vi "createColorProjections.vi"(4 "xyz order":bool, 6 "max values":T2={"xy max"={"r max"=-1.0, "g max"=-1.0, "b max"=-1.0}, "xz max"={"r max"=-1.0, "g max"=-1.0, "b max"=-1.0}, "zy max"={"r max"=-1.0, "g max"=-1.0, "b max"=-1.0}}, 7 "display channels":cluster{"CH0":bool, "CH1":bool}, 8 "error in (no error)":errorcluster, 9 "spilt ff/fb":bool, 10 "color ims":cluster{"xy im":T3, "xz im":T3, "yz im":T3}, 11 "volumes for display":T5) -> (0 "error out":errorcluster, 1 "deltaZ":dbl, 2 "pixel sums":cluster{"ch0 sum":u32, "ch1 sum":u32}, 3 "color ims out":T4, 5 "max values from im":T1)   [LabVIEW 2010]
uses:
  <vilib>/vision/Image Controls.llb/IMAQ Image.ctl
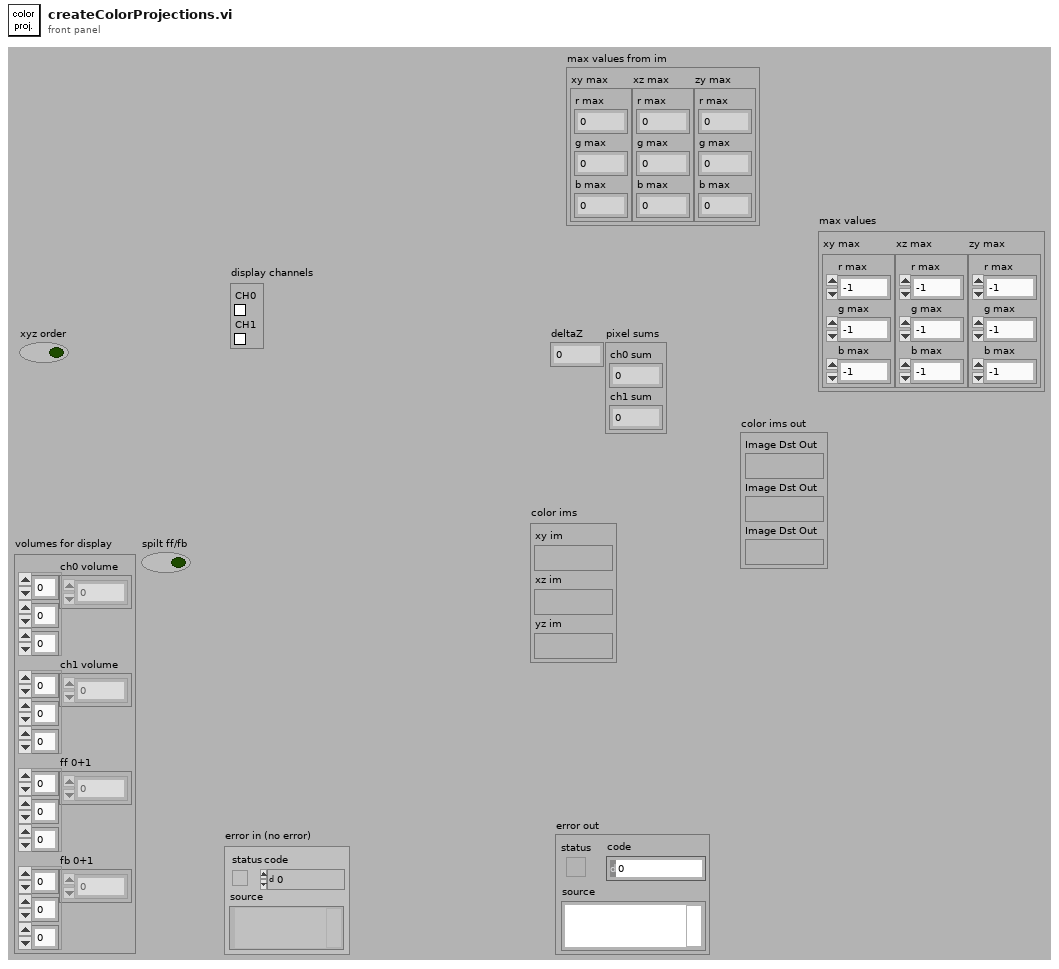
[diagram p1: front panel]
types:
  T1 = cluster{"xy max":cluster{"r max":u32, "g max":u32, "b max":u32}, "xz max":cluster{"r max":u32, "g max":u32, "b max":u32}, "zy max":cluster{"r max":u32, "g max":u32, "b max":u32}}
  T2 = cluster{"xy max":cluster{"r max":dbl, "g max":dbl, "b max":dbl}, "xz max":cluster{"r max":dbl, "g max":dbl, "b max":dbl}, "zy max":cluster{"r max":dbl, "g max":dbl, "b max":dbl}}
  T3 = typedef "IMAQ Image.ctl" = refnum<image>
  T4 = cluster{"Image Dst Out":T3, "Image Dst Out":T3, "Image Dst Out":T3}
  T5 = cluster{"ch0 volume":u32[][][], "ch1 volume":u32[][][], "ff 0+1":u32[][][], "fb 0+1":u32[][][]}
  T6 = cluster{"max vals from im":cluster{"r max":u32, "g max":u32, "b max":u32}, "max vals from im":cluster{"r max":u32, "g max":u32, "b max":u32}, "max vals from im":cluster{"r max":u32, "g max":u32, "b max":u32}}
  T7 = cluster{"Image Out":T3, "Image Out":T3, "Image Out":T3}
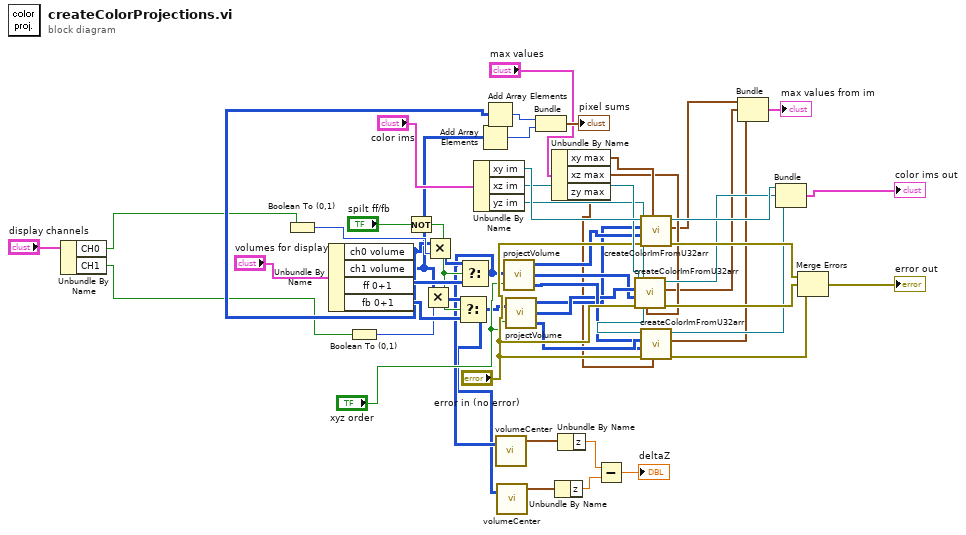
[diagram p0: block diagram]
diagram:
  n1 = Unbundle By Name("display channels") -> ("CH0"=w2:bool, "CH1"=w1:bool)
  n2 = Boolean To (0,1)(Boolean=w2) -> (0, 1=w33:i16)
  n3 = Unbundle By Name("volumes for display") -> ("ch0 volume"=w16:u32[][][], "ch1 volume"=w15:u32[][][], "ff 0+1"=w50:u32[][][], "fb 0+1"=w47:u32[][][])
  n4 = Boolean To (0,1)(Boolean=w1) -> (0, 1=w31:i16)
  n5 = Not(x="spilt ff/fb") -> (.not. x?=w48:bool)
  n6 = Multiply(x=w15, y=w31) -> (x*y=w32:u32[][][])
  n7 = Multiply(x=w16, y=w33) -> (x*y=w34:u32[][][])
  n8 = Select(t=w32, s=w48, f=w47) -> (s? t:f=w28:u32[][][])
  n9 = Select(t=w34, s=w48, f=w50) -> (s? t:f=w29:u32[][][])
  n10 = Unbundle By Name("color ims") -> ("xy im"=w45:T3, "xz im"=w44:T3, "yz im"=w43:T3)
  n11 = Add Array Elements(numeric array=w15) -> (sum=w13:u32)
  n12 = Add Array Elements(numeric array=w16) -> (sum=w14:u32)
  n13 = call "volumeCenter.vi"("input array"=w29) -> ("mean location"=w27:cluster{"x":dbl, "y":dbl, "z":dbl})  [unwired: 3 in]
  n14 = call "volumeCenter.vi"("input array"=w28) -> ("mean location"=w26:cluster{"x":dbl, "y":dbl, "z":dbl})  [unwired: 3 in]
  n15 = call "projectVolume.vi"("xyz order"="xyz order", "input array"=w29) -> ("ZY view"=w21:u32[][], "XZ view"=w19:u32[][], "XY view"=w18:u32[][])
  n16 = call "projectVolume.vi"("xyz order"="xyz order", "input array"=w28) -> ("ZY view"=w22:u32[][], "XZ view"=w20:u32[][], "XY view"=w17:u32[][])
  n17 = Bundle("Numeric"=w14, "Numeric"=w13) -> (→"pixel sums":cluster{"Numeric":u32, "Numeric":u32})  [unwired: 1 in]
  n18 = Unbundle By Name("max values") -> ("xy max"=w10:cluster{"r max":dbl, "g max":dbl, "b max":dbl}, "xz max"=w9:cluster{"r max":dbl, "g max":dbl, "b max":dbl}, "zy max"=w8:cluster{"r max":dbl, "g max":dbl, "b max":dbl})
  n19 = Unbundle By Name(w26) -> ("z"=w25:dbl)
  n20 = Unbundle By Name(w27) -> ("z"=w24:dbl)
  n21 = Subtract(x=w24, y=w25) -> (x-y=→"deltaZ":dbl)
  n22 = call "createColorImFromU32arr.vi"("max vals (-1 for autoscale)"=w9, "error in (no error)"="error in (no error)", "g buffer"=w19, "r buffer"=w20, "Image"=w44) -> ("error out"=w41:errorcluster, "max vals from im"=w6:cluster{"r max":u32, "g max":u32, "b max":u32}, "Image Out"=w38:T3)  [unwired: 4 in]
  n23 = call "createColorImFromU32arr.vi"("max vals (-1 for autoscale)"=w10, "error in (no error)"="error in (no error)", "g buffer"=w18, "r buffer"=w17, "Image"=w45) -> ("error out"=w42:errorcluster, "max vals from im"=w7:cluster{"r max":u32, "g max":u32, "b max":u32}, "Image Out"=w39:T3)  [unwired: 4 in]
  n24 = call "createColorImFromU32arr.vi"("max vals (-1 for autoscale)"=w8, "error in (no error)"="error in (no error)", "g buffer"=w21, "r buffer"=w22, "Image"=w43) -> ("error out"=w40:errorcluster, "max vals from im"=w5:cluster{"r max":u32, "g max":u32, "b max":u32}, "Image Out"=w37:T3)  [unwired: 4 in]
  n25 = Bundle("max vals from im"=w7, "max vals from im"=w6, "max vals from im"=w5) -> (→"max values from im":T6)  [unwired: 1 in]
  n26 = Bundle("Image Out"=w39, "Image Out"=w38, "Image Out"=w37) -> (→"color ims out":T7)  [unwired: 1 in]
  n27 = Merge Errors(w42, w41, w40) -> (→"error out":errorcluster)
